vi "VAttrbutes-Merge.vi"(6 "If exist? Skip(T)/Overwrite(F)":bool, 8 "error in (no error)":errorcluster, 10 "VAttributes B":variant, 11 "VAttributes A":variant) -> (0 "error out":errorcluster, 3 "VAttributes A after B->A":variant)   [LabVIEW 2019]
uses:
  <userlib>/_OpenG.lib/lvdata/lvdata.llb/Get Data Name__ogtk.vi
  <userlib>/NEVSTOP-Programming-Palette/Configuration/ClusterCfgTable/Indexed String To Enum_nevstop.vi
  <userlib>/_OpenG.lib/error/error.llb/Build Error Cluster__ogtk.vi
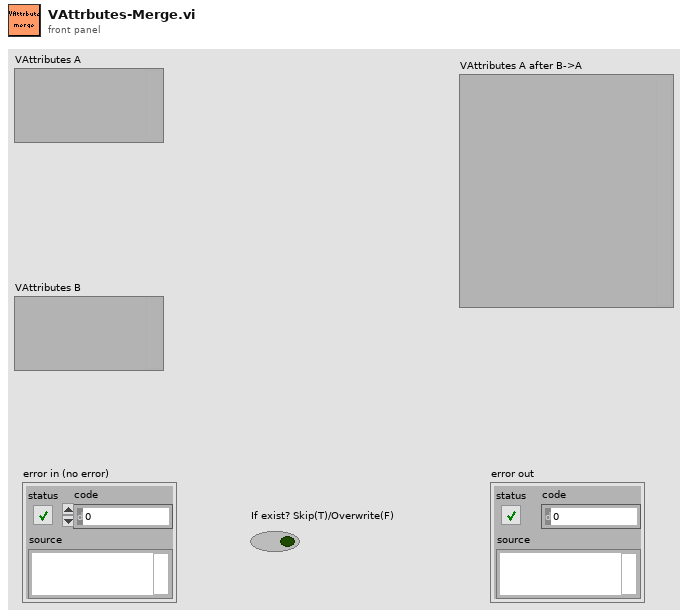
[diagram p1: front panel]
types:
  T1 = typedef "Type Descriptor Enumeration__ogtk.ctl" = enum8{"<Null>", "I8", "I16", "I32", "I64", "U8", "U16", "U32", "U64", "SGL", "DBL", "EXT", "CSG", "CDB", "CXT", "0x0F", "0x10", "0x11", "0x12", "0x13", "0x14", "Enum U8", "Enum U16", "Enum U32", "Enum U64", "SGL PQ", "DBL PQ", "EXT PQ", "CSG PQ", "CDB PQ", "CXT PQ", "0x1F", "0x20", "Boolean", "0x22", "0x23", "0x24", "0x25", "0x26", "0x27", "0x28", "0x29", "0x2A", "0x2B", "0x2C", "0x2D", "0x2E", "0x2F", "String", "0x31", "Path", "Pict", "0x34", "0x35", "0x36", "DAQ", "0x38", "0x39", "0x3A", "0x3B", "0x3C", "0x3D", "0x3E", "0x3F", "Array", "0x41", "0x42", "0x43", "0x44", "0x45", "0x46", "0x47", "0x48", "0x49", "0x4A", "0x4B", "0x4C", "0x4D", "0x4E", "0x4F", "Cluster", "0x51", "0x52", "Variant", "Waveform", "0x55", "0x56", "0x57", "0x58", "0x59", "0x5A", "0x5B", "0x5C", "0x5D", "0x5E", "0x5F", "0x60", "0x61", "0x62", "0x63", "0x64", "0x65", "0x66", "0x67", "0x68", "0x69", "0x6A", "0x6B", "0x6C", "0x6D", "0x6E", "0x6F", "Refnum"}
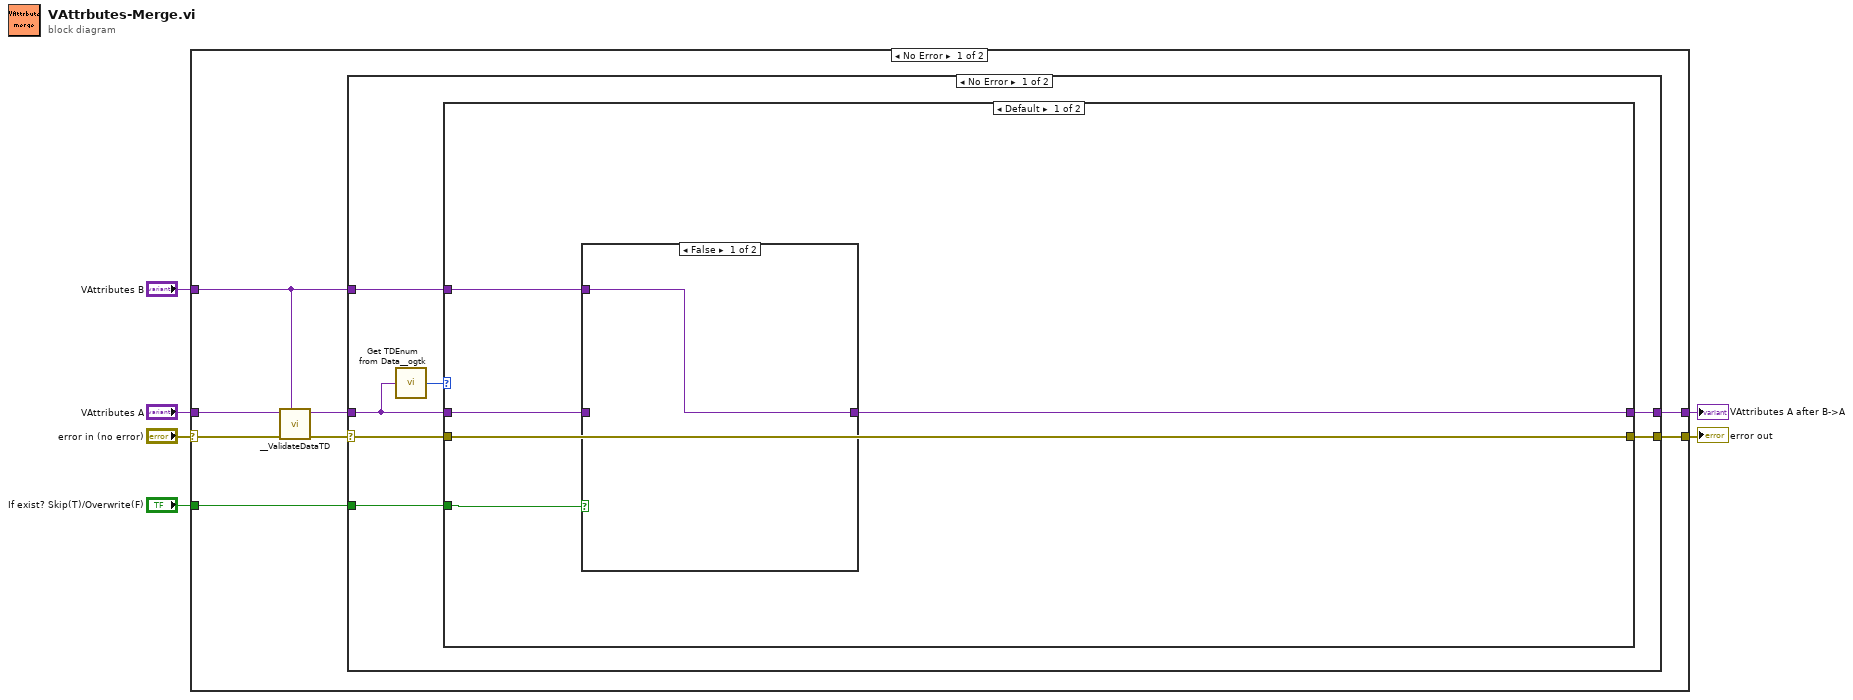
[diagram p0: block diagram]
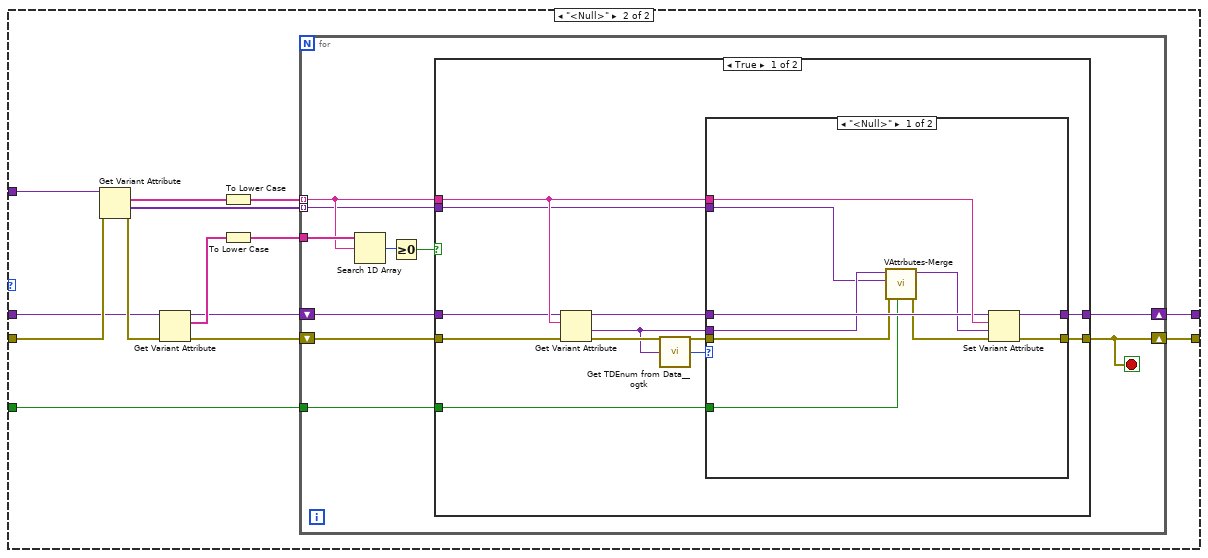
[diagram p3: hidden frame]
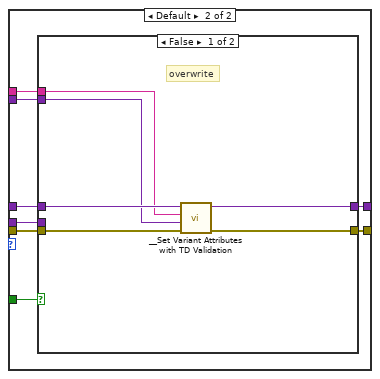
[diagram p4: hidden frame]
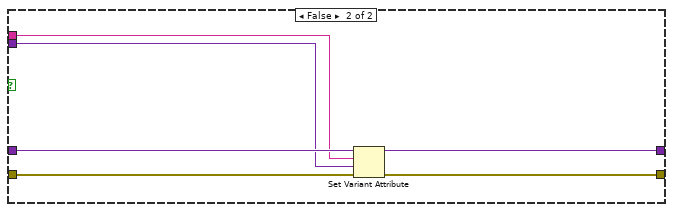
[diagram p6: hidden frame]
diagram:
  n1 = case shown="No Error" "error in (no error)" {
    selector: "error in (no error)" -> [w8 w99]
    tunnel: "VAttributes A" -> [w11 w98]
    tunnel: "VAttributes B" -> [w7 _]
    tunnel: "If exist? Skip(T)/Overwrite(F)" -> [w12 _]
    tunnel: [w13 w99] -> w2
    tunnel: [w14 w98] -> w1
    frame No Error {
      n2 = call "__ValidateDataTD.vi"("Expected Data"=w7, "error in (no error)"=w8, "Data"=w11) -> ("error out"=w9:errorcluster, "Data out"=w10:variant)  [unwired: 7 in]
      n3 = case shown="No Error" w9 {
        selector: w9 -> [w19 w96]
        tunnel: [w21 w97] -> w14
        tunnel: [w20 w96] -> w13
        tunnel: w12 -> [w17 _]
        tunnel: w7 -> [w18 _]
        tunnel: w10 -> [w15 w97]
        frame No Error {
          n4 = call <userlib>:"Get TDEnum from Data__ogtk.vi"("Data"=w15) -> ("Type Descriptor Enumeration"=w16:T1)  [unwired: 4 in]
          n5 = case shown="Default" w16 {
            tunnel: [w23 w34] -> w21
            tunnel: [w26 w33] -> w20
            tunnel: w19 -> [w26 w32]
            tunnel: w15 -> [w24 w31]
            tunnel: w18 -> [w22 w30]
            tunnel: w17 -> [w25 w29]
            frame Default {
              n6 = case shown="False" w25 {
                tunnel: w24 -> [_ w28]
                tunnel: [w27 w28] -> w23
                tunnel: w22 -> [w27 _]
                frame False {
                }
                frame True {
                }
              }
            }
            frame "<Null>" {
              n7 = Get Variant Attribute(Variant=w30, error in=w32) -> (names=w40:string[], values=w39:variant[], error out=w38:errorcluster)  [unwired: 2 in, 1 out]
              n8 = Get Variant Attribute(Variant=w31, error in=w38) -> (duplicate Variant=w35:variant, names=w36:string[], error out=w42:errorcluster)  [unwired: 2 in, 1 out]
              n9 = To Lower Case(string=w40) -> (all lower case string=w41:string[])
              n10 = To Lower Case(string=w36) -> (all lower case string=w37:string[])
              n11 = for {
                shift-right: [w51] -> w34
                shift-left: w35 -> [w52]
                shift-right: [w43] -> w33
                shift-left: w42 -> [w50]
                tunnel: w37 -> [w49]
                tunnel: w39 -> [w45] mode=indexing
                tunnel: w41 -> [w46] mode=indexing
                tunnel: w29 -> [w44]
                stop <- w43 stop-if-true
                n12 = Search 1D Array(1D array=w49, element=w46) -> (index of element=w48:i32)  [unwired: 1 in]
                n13 = Greater Or Equal To 0?(x=w48) -> (x >= 0?=w47:bool)
                n14 = case shown="True" w47 {
                  tunnel: w52 -> [w58 w95]
                  tunnel: [w63 w94] -> w51
                  tunnel: w50 -> [w62 w93]
                  tunnel: [w61 w92] -> w43
                  tunnel: w46 -> [w60 w91]
                  tunnel: w45 -> [w55 w90]
                  tunnel: w44 -> [w57 _]
                  frame True {
                    n15 = Get Variant Attribute(Variant=w58, name=w60, error in=w62) -> (duplicate Variant=w59:variant, value=w54:variant, error out=w56:errorcluster)  [unwired: 1 in, 1 out]
                    n16 = call <userlib>:"Get TDEnum from Data__ogtk.vi"("Data"=w54) -> ("Type Descriptor Enumeration"=w53:T1)  [unwired: 4 in]
                    n17 = case shown="\"<Null>\"" w53 {
                      tunnel: [w73 w81] -> w63
                      tunnel: [w72 w78] -> w61
                      tunnel: w60 -> [w71 w79]
                      tunnel: w59 -> [w70 w76]
                      tunnel: w55 -> [w68 w77]
                      tunnel: w54 -> [w69 w74]
                      tunnel: w56 -> [w67 w80]
                      tunnel: w57 -> [w64 w75]
                      frame "<Null>" {
                        n18 = call "VAttrbutes-Merge.vi"("If exist? Skip(T)/Overwrite(F)"=w64, "error in (no error)"=w67, "VAttributes B"=w68, "VAttributes A"=w69) -> ("error out"=w66:errorcluster, "VAttributes A after B->A"=w65:variant)  [unwired: 6 in]
                        n19 = Set Variant Attribute(Variant=w70, name=w71, value=w65, error in=w66) -> (Variant out=w73:variant, error out=w72:errorcluster)  [unwired: 1 out]
                      }
                      frame Default {
                        n20 = case shown="False" w75 {
                          tunnel: [w87 w89] -> w81
                          tunnel: w80 -> [w86 w88]
                          tunnel: w79 -> [w82 _]
                          tunnel: [w85 w88] -> w78
                          tunnel: w77 -> [w83 _]
                          tunnel: w76 -> [w84 w89]
                          tunnel: w74 -> [_ _]
                          frame False {
                            # "overwrite"
                            n21 = call "__Set Variant Attributes with TD Validation.vi"("error in (no error)"=w86, "data"=w83, "String"=w82, "Map"=w84) -> ("error out"=w85:errorcluster, "Map"=w87:variant)  [unwired: 6 in]
                          }
                          frame True {
                            # "Skip"
                          }
                        }
                      }
                    }
                  }
                  frame False {
                    n22 = Set Variant Attribute(Variant=w95, name=w91, value=w90, error in=w93) -> (Variant out=w94:variant, error out=w92:errorcluster)  [unwired: 1 out]
                  }
                }
              }
            }
          }
        }
        frame Error {
        }
      }
    }
    frame Error {
    }
  }
  "error out" <- w2
  "VAttributes A after B->A" <- w1
